vi "MakeRoom.vi"(8 "error in (no error)":errorcluster, 10 "RoomNumber":i32, 11 "BombedMazeGame":refnum<class "BombedMazeGame.lvclass">) -> (0 "error out":errorcluster, 2 "Room":refnum<class "Room.lvclass">, 3 "BombedMazeGame":refnum<class "BombedMazeGame.lvclass">)   [LabVIEW 2020, in "FactoryMethod.lvlib" / "NoParametrizedFactoryMethod.lvlib" / "BombedMazeGame.lvclass"]
uses:
  BombedMazeGame.lvclass
  GoFcommonClasses/ConcreteMazeSite/Room/Room.lvclass
  GoFcommonClasses/ConcreteMazeSite/RoomWithBomb/RoomWithBomb.lvclass
  E:/Francesco/GitHub/Design-Patterns-GoF_-_NI-LV/Creational/GoFcommonClasses/ConcreteMazeSite/Room/Room.lvclass
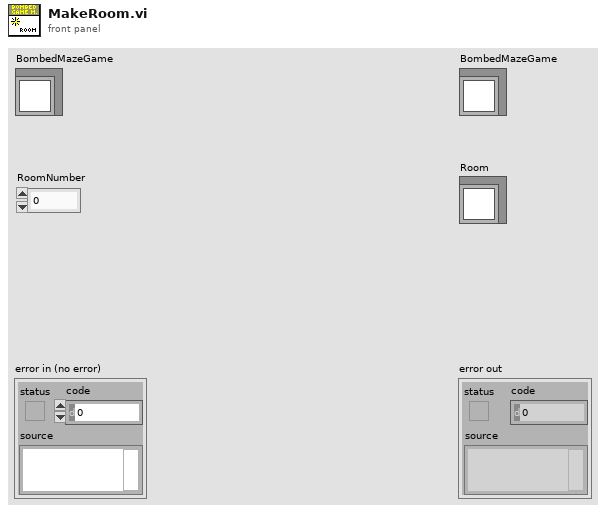
[diagram p1: front panel]
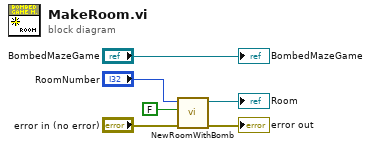
[diagram p0: block diagram]
diagram:
  n1 = call "NewRoomWithBomb.vi"("error in (no error)"="error in (no error)", "Bombed"=FALSE, "RoomNumber"="RoomNumber") -> ("error out"=→"error out":errorcluster, "RoomWithBomb"=→"Room":refnum<class "RoomWithBomb.lvclass">)  [unwired: 7 in]
  "BombedMazeGame" <- "BombedMazeGame"
